vi "Is In SubPanel.vi"(8 "error in (no error)":errorcluster, 10 "Panel":refnum<class "Panel.lvclass">, 11 "PanelManager in":refnum<class "PanelManager.lvclass">) -> (0 "error out":errorcluster, 2 "In SubPanel?":bool, 3 "PanelManager out":refnum<class "PanelManager.lvclass">)   [LabVIEW 2018, in "OOPanel.lvlib" / "PanelManager.lvclass"]
uses:
  PanelManager.lvclass
  Panel/Panel.lvclass
  PanelManager.lvclass/PanelManager.ctl
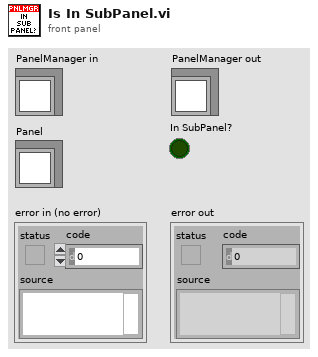
[diagram p1: front panel]
types:
  T1 = typedef "OOPanel.lvlib/PanelManager.lvclass/Ref Data.ctl" = cluster{"Panels":T2, "Subpanel Map":T3}
  T2 = typedef "OOPanel.lvlib/PanelManager.lvclass/Panels.ctl" = cluster{"Names":string[], "Instances":refnum<class "Panel.lvclass">[]}
  T3 = typedef "OOPanel.lvlib/PanelManager.lvclass/SubPanel Map.ctl" = cluster{"SubPanels":refnum<vi>[], "Panels":refnum<class "Panel.lvclass">[]}
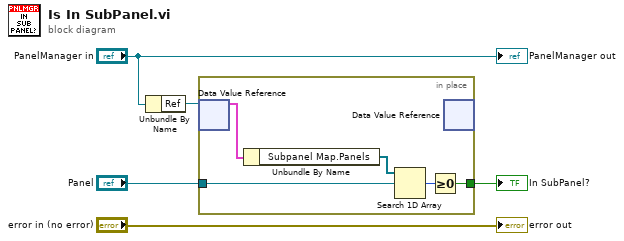
[diagram p0: block diagram]
diagram:
  n1 = Unbundle By Name("PanelManager in") -> ("Ref"=w3:refnum<data-value>)
  n2 = in-place {
    in-place-border: "Panel" -> [w9]
    in-place-border: [w6] -> w1
    n3 = in-place-dvr #1(w3) -> (w10:T1)  [unwired: 1 out]
    n4 = Unbundle By Name(w10) -> ("Subpanel Map.Panels"=w8:refnum<class "Panel.lvclass">[])
    n5 = Search 1D Array(1D array=w8, element=w9) -> (index of element=w7:i32)  [unwired: 1 in]
    n6 = Greater Or Equal To 0?(x=w7) -> (x >= 0?=w6:bool)
    n7 = in-place-dvr #1() -> ()  [unwired: 1 in, 2 out]
  }
  "In SubPanel?" <- w1
  "error out" <- "error in (no error)"
  "PanelManager out" <- "PanelManager in"
